vi "4-ConnectPLC.vi"(8 "error in (no error)":errorcluster, 11 "AllControls In":T1) -> ()   [LabVIEW 2017]
uses:
  Ctrls/AlarmIndex.ctl
  Ctrls/AllControls.ctl
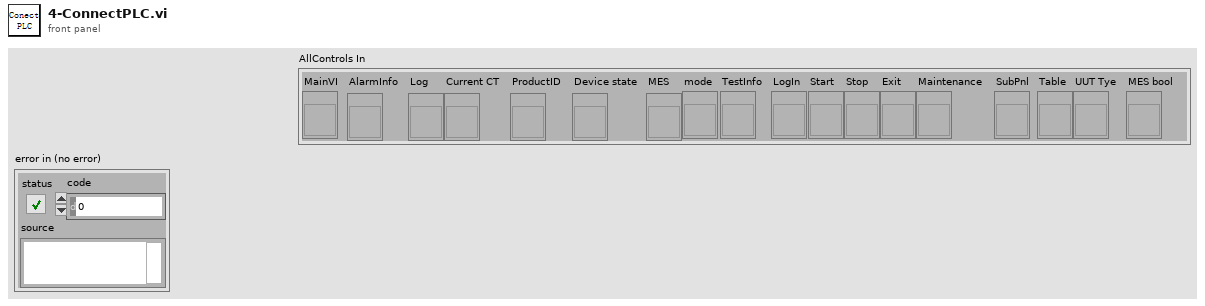
[diagram p1: front panel]
types:
  T1 = typedef "AllControls.ctl" = cluster{"MainVI":refnum<vi>, "AlarmInfo":refnum<vi>, "Log":refnum<vi>, "Current CT":refnum<vi>, "ProductID":refnum<vi>, "Device state":refnum<vi>, "MES":refnum<vi>, "mode":refnum<vi>, "TestInfo":refnum<vi>, "LogIn":refnum<vi>, "Start":refnum<vi>, "Stop":refnum<vi>, "Exit":refnum<vi>, "Maintenance":refnum<vi>, "SubPnl":refnum<vi>, "Table":refnum<vi>, "UUT Tye":refnum<vi>, "MES bool":refnum<vi>}
  T2 = typedef "AlarmIndex.ctl" = enum16{"The security grating is triggered", "The safety door is open", "Upper servo motor alarm", "Left servo motor alarm", "Right servo motor alarm", "The upper servo motor exceeds the pressure", "The left servo motor exceeds the pressure", "The right servo motor exceeds the pressure", "Emergency trigger", "Open VISA Error,Please check the serial port", "PLC UDP Error,Please check the network", "Scanner connect Error,Please check the network", "D620 Error,Please check"}
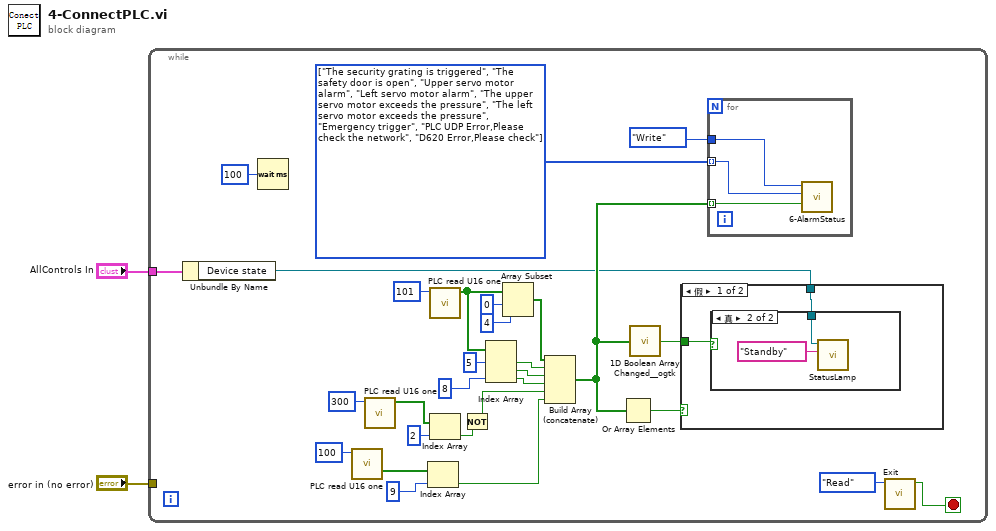
[diagram p0: block diagram]
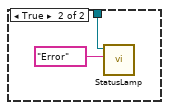
[diagram p4: hidden frame]
diagram:
  n1 = while {
    tunnel: "AllControls In" -> [w4]
    tunnel: "error in (no error)" -> [_]
    stop <- w30 stop-if-true
    w16 = T2[] [enum."The security grating is triggered", enum."The safety door is open", enum."Upper servo motor alarm", enum."Left servo motor alarm", enum."The upper servo motor exceeds the pressure", enum."The left servo motor exceeds the pressure", enum."Emergency trigger", enum."PLC UDP Error,Please check the network", enum."D620 Error,Please check"] items=["The security grating is triggered", "The safety door is open", "Upper servo motor alarm", "Left servo motor alarm", "Right servo motor alarm", "The upper servo motor exceeds the pressure", "The left servo motor exceeds the pressure", "The right servo motor exceeds the pressure", "Emergency trigger", "Open VISA Error,Please check the serial port", "PLC UDP Error,Please check the network", "Scanner connect Error,Please check the network", "D620 Error,Please check"]
    n2 = Unbundle By Name(w4) -> ("Device state"=w3:refnum<vi>)
    n3 = Wait (ms)(milliseconds to wait=u32 100) -> ()  [unwired: 1 out]
    n4 = call "PLC read U16 one.vi"("Address"=u16 100) -> ("Data"=w10:bool[])  [unwired: 8 in, 1 out]
    n5 = call "PLC read U16 one.vi"("Address"=u16 300) -> ("Data"=w19:bool[])  [unwired: 8 in, 1 out]
    n6 = Index Array(array=w10, index=9) -> (element=w8:bool)
    n7 = call "PLC read U16 one.vi"("Address"=u16 101) -> ("Data"=w23:bool[])  [unwired: 8 in, 1 out]
    n8 = Index Array(array=w19, index=2) -> (element=w18:bool)
    n9 = Not(x=w18) -> (.not. x?=w17:bool)
    n10 = Index Array(array=w23, index #1=5 ("index"), index #3=8 ("index")) -> (element #1=w22:bool, element #2=w13:bool, element #3=w12:bool)  [unwired: 1 in]
    n11 = Array Subset(array=w23, index=0, length=4) -> (w26:bool[])
    n12 = Build Array (concatenate)(w26, w22, w13, w12, w17, w8) -> (w7:bool[])
    n13 = Or Array Elements(Boolean array=w7) -> (logical OR=w6:bool)
    n14 = call "1D Boolean Array Changed__ogtk.vi"("1D Boolean Array"=w7) -> ("Changed"=w5:bool)
    n15 = case shown="假" w6 {
      tunnel: w5 -> [w33 w37]
      tunnel: w3 -> [w32 w36]
      frame False {
        n16 = case shown="真" w33 {
          tunnel: w32 -> [_ w34]
          frame False {
          }
          frame True {
            n17 = call "StatusLamp.vi"("State"="Standby", "Boolean输入"=w34) -> ()  [unwired: 9 in, 1 out]
          }
        }
      }
      frame True {
        n18 = case shown="假" w37 {
          tunnel: w36 -> [_ w39]
          frame False {
          }
          frame True {
            n19 = call "StatusLamp.vi"("State"="Error", "Boolean输入"=w39) -> ()  [unwired: 9 in, 1 out]
          }
        }
      }
    }
    n20 = for {
      tunnel: w7 -> [w42] mode=indexing
      tunnel: w16 -> [w41] mode=indexing
      tunnel: enum16{"Initial", "Write", "Read"}."Write" ("Step") -> [w40]
      n21 = call "6-AlarmStatus.vi"("AlarmValue"=w42, "AlarmIndex"=w41, "Step"=w40) -> ()  [unwired: 7 in, 2 out]
    }
    n22 = call "Exit.vi"("Step"=enum16{"Initial", "Write", "Read"}."Read" ("step")) -> ("Exit Out"=w30:bool)  [unwired: 9 in, 1 out]
  }
